vi "Rayon max.vi"(10 "Capteur 3 ou 4":dbl[](array[numeric]), 11 "Capteur 2":dbl[](array[numeric])) -> (3 "Rayon max":dbl)   [LabVIEW 2018]
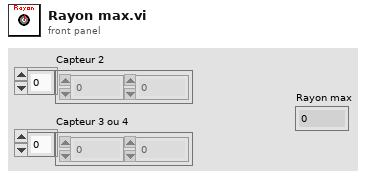
[diagram p1: front panel]
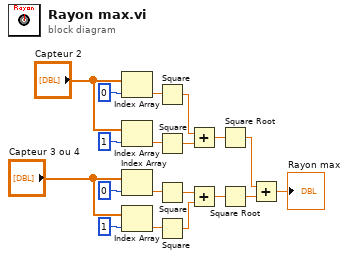
[diagram p0: block diagram]
diagram:
  n1 = Index Array(array="Capteur 2", index=0 ("indice")) -> (element=w15:dbl)
  n2 = Index Array(array="Capteur 2", index=1 ("indice")) -> (element=w16:dbl)
  n3 = Index Array(array="Capteur 3 ou 4", index=0 ("indice")) -> (element=w8:dbl)
  n4 = Index Array(array="Capteur 3 ou 4", index=1 ("indice")) -> (element=w9:dbl)
  n5 = Square(x=w15) -> (x^2=w13:dbl)
  n6 = Square(x=w16) -> (x^2=w14:dbl)
  n7 = Square(x=w8) -> (x^2=w6:dbl)
  n8 = Square(x=w9) -> (x^2=w7:dbl)
  n9 = Add(x=w13, y=w14) -> (x+y=w12:dbl)
  n10 = Add(x=w6, y=w7) -> (x+y=w5:dbl)
  n11 = Square Root(x=w12) -> (sqrt(x)=w3:dbl)
  n12 = Square Root(x=w5) -> (sqrt(x)=w2:dbl)
  n13 = Add(x=w3, y=w2) -> (x+y=→"Rayon max":dbl)
